vi "Grab and Broadcast (Controller).vi"() -> ()   [LabVIEW 2011]
doc: "The Grab and Broadcast (Controller) VI acquires images continuously and displays the images in an image control using high-level acquisition VIs. This VI also demonstrates camera control in a broadcasting application. A grab is appropriate for high-speed applications in which you need to process only one image at a time."
uses:
  <vilib>/vision/driver/NI_Vision_Acquisition_Software.lvlib
  <vilib>/vision/driver/IMAQdx.llb/IMAQdx Camera Control Mode.ctl
panel:
  in  "Camera Name":refnum<k21> caption="IMAQdx Session"
  out "Buffer Number":u32
  out "Image":T1(plugin-control)
  out "Frame Rate":dbl(knob) scale=0.0..100.0
  in  "Stop":bool
  # "Overview: Demonstrates how to broadcast images so multiple machines can acquire the same images from a camera.\nRequirements: Vision Acquisition Software\nInstructions: \n1. Select the Camera Name \n2. Run the Grab and Broadcast (Controller) VI.\n3. On a different machine or target, run the Grab and Broadcast (Listener) VI using the same camera."
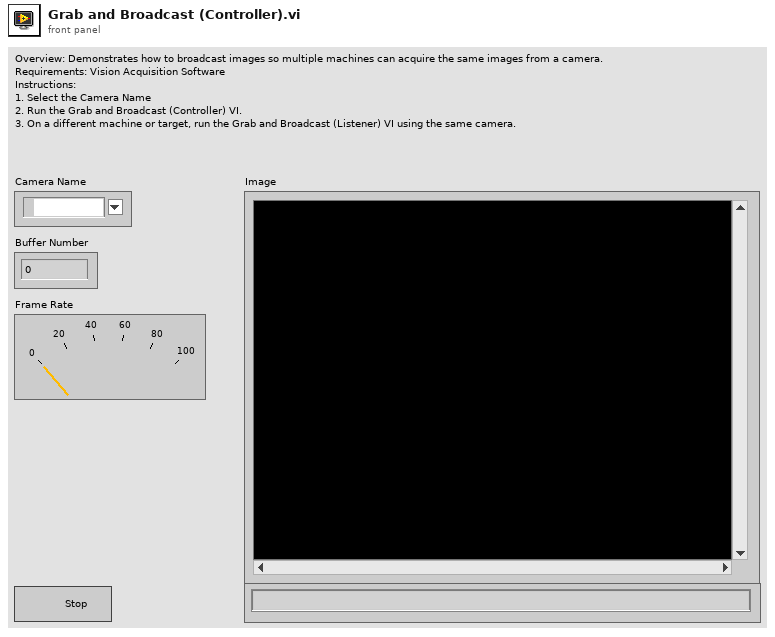
[diagram p1: front panel]
types:
  T1 = typedef "IMAQ Image.ctl" = refnum<image>
  T2 = typedef "NI_Vision_Acquisition_Software.lvlib/IMAQdx Camera Control Mode.ctl" = enum32{"Controller", "Listener"}
  T3 = typedef "IMAQdx.ctl" = refnum<k21>
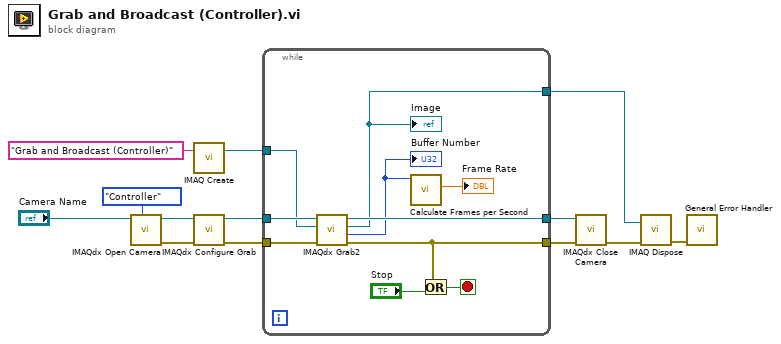
[diagram p0: block diagram]
diagram:
  n1 = call <vilib>:"IMAQdx Open Camera.vi"("Camera Control Mode"=IMAQdx_Camera_Control_Mode."Controller", "Session In"="Camera Name") -> ("error out"=w9:errorcluster, "Session Out"=w10:T3)  [unwired: 1 in, 7 out]
  n2 = call "IMAQ Create"("Image Name"="Grab and Broadcast (Controller)") -> ("New Image"=w13:T1)  [unwired: 3 in, 2 out]
  n3 = call <vilib>:"IMAQdx Configure Grab.vi"("error in"=w9, "Session In"=w10) -> ("error out"=w1:errorcluster, "Session Out"=w2:T3)  [unwired: 8 out]
  n4 = while {
    tunnel: [w19] -> w12
    tunnel: w1 -> [w21]
    tunnel: w2 -> [w22]
    tunnel: [w16] -> w11
    tunnel: w13 -> [w20]
    tunnel: [w14] -> w3
    stop <- w23 stop-if-true
    n5 = call <vilib>:"IMAQdx Grab2.vi"("error in"=w21, "Image In"=w20, "Session In"=w22) -> ("error out"=w16:errorcluster, "Buffer Number Out"=w17:u32, "Image Out"=w14:T1, "Session Out"=w19:T3)  [unwired: 5 in]
    "Image" <- w14
    "Buffer Number" <- w17
    n6 = call <vilib>:"Calculate Frames per Second.vi"("Buffer Number"=w17) -> ("Processed Frames/s"=→"Frame Rate":dbl)  [unwired: 8 in, 2 out]
    n7 = Or(x=w16, y="Stop") -> (x .or. y?=w23:bool)
  }
  n8 = call <vilib>:"IMAQdx Close Camera.vi"("error in"=w11, "Session In"=w12) -> ("error out"=w5:errorcluster)  [unwired: 9 out]
  n9 = call "IMAQ Dispose"("Image"=w3, "error in (no error)"=w5) -> ("error out"=w4:errorcluster)  [unwired: 4 in]
  n10 = call <vilib>:"General Error Handler.vi"("error in (no error)"=w4) -> ()  [unwired: 1 in, 14 out]
